vi "Library Extract String Lines.vi"(7 "multi-line string":string) -> (8 "lines":string[](array[string]))   [LabVIEW 2012]
doc: "Extract the lines from a multi-line string and returns them as an array of lines excluding line terminators. It considers the line terminators of the various platforms (\\n, \\r\\n, and \\r) as valid line endings."
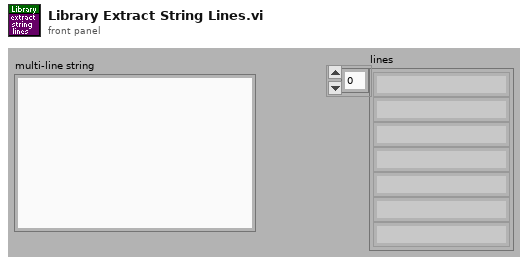
[diagram p1: front panel]
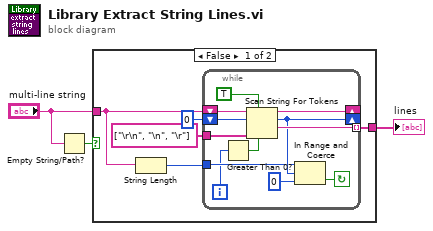
[diagram p0: block diagram]
diagram:
  n1 = Empty String/Path?(string/path="multi-line string") -> (empty?=w1:bool)
  n2 = case shown="False" w1 {
    tunnel: "multi-line string" -> [w6 _]
    tunnel: [w5 _] -> w3
    frame False {
      n3 = String Length(string=w6) -> (length=w4:i32)
      n4 = while {
        shift-right: [w19] -> _
        shift-left: w6 -> [w20]
        tunnel: string[] ["\r\n", "\n", "\r"] ("delimiters (\\s,\\t,\\r,\\n)") -> [w18]
        shift-right: [w15] -> _
        shift-left: 0 ("offset past token") -> [w17]
        tunnel: [w16] -> w5 mode=indexing
        tunnel: w4 -> [w13]
        i -> [w10]
        stop <- w12 continue-if-true
        n5 = Greater Than 0?(x=w10) -> (x > 0?=w11:bool)
        n6 = Scan String For Tokens(4:w11, 5:TRUE ("allow empty tokens? (F)"), 6:w18, 8:w17, 9:w20) -> (1:w16:string, 2:w15:i32, 3:w19:string)  [unwired: 1 in, 1 out]
        n7 = In Range and Coerce(upper limit=w13, x=w15, lower limit=0) -> (In Range?=w12:bool)  [unwired: 1 out]
      }
    }
    frame True {
    }
  }
  "lines" <- w3
